vi "Receive Event with Logging.vi"(6 "Global Log Level":T1, 7 "Mediated Actor in":refnum<class "Mediated Actor.lvclass">, 8 "error in (no error)":errorcluster, 11 "Message":refnum<class "Message Interface.lvclass">) -> (0 "error out":errorcluster, 2 "Name":string, 3 "Message out":refnum<class "Message Interface.lvclass">, 5 "Mediated Actor out":refnum<class "Mediated Actor.lvclass">)   [LabVIEW 2016, in "Stream Mediator.lvlib" / "Mediated Actor.lvclass"]
doc: "--\nCopyright © 2017 Composed SystemsI All rights reserved.\n\nAuthor: Jon McBee <jon.mcbee@composed.io>\n\nThis library is provided \"AS IS\" ,WITHOUT WARRANTIES OR\nCONDITIONS OF ANY KIND, either express or implied.\n\nComposed Systems -- composed.io\n\nStream 0.0.1.1\nJon McBee - Composed Systems\nCopyright (c) 2017, Composed Systems"
uses:
  <userlib>/Composed Systems/Stream/Mediator/Classes/Mediated Actor/Mediated Actor.lvclass
  C:/Program Files (x86)/National Instruments/LabVIEW 2016/user.lib/Composed Systems/Stream/Actor/Actor Class/Ancestral Actor.lvclass
  <userlib>/Composed Systems/Stream/Mediator/Classes/Message Interface/Message Interface.lvclass
  <userlib>/Composed Systems/Stream/Log/Application Log/Log Level.ctl
  <userlib>/Composed Systems/Stream/Actor/Actor Class/Ancestral Actor.lvclass/Ancestral Actor.ctl
  <userlib>/Composed Systems/Stream/Mediator/Classes/Message Interface/Message Interface.lvclass/Message Interface.ctl
  <userlib>/Composed Systems/Stream/Log/Global Application Log/Global Application Log.lvclass
  <userlib>/Composed Systems/Stream/Actor/Actor Class/Ancestral Actor.lvclass
  <userlib>/Composed Systems/Stream/Log/Application Log/Application Log.lvclass
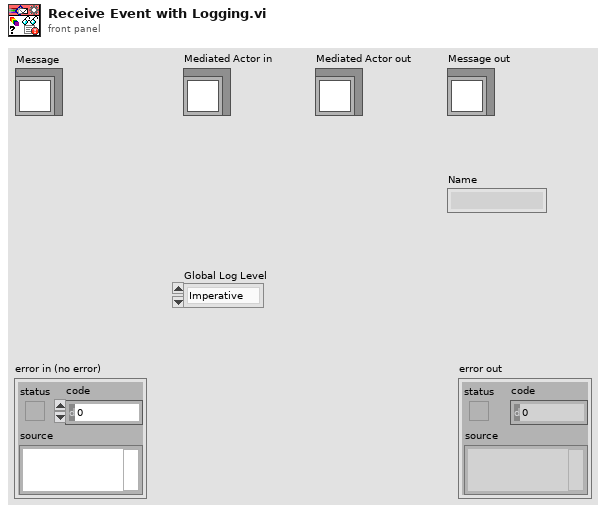
[diagram p1: front panel]
types:
  T1 = typedef "Stream Log.lvlib/Application Log.lvclass/Log Level.ctl" = enum16{"Imperative", "Major", "Minor", "Debug", "Off"}
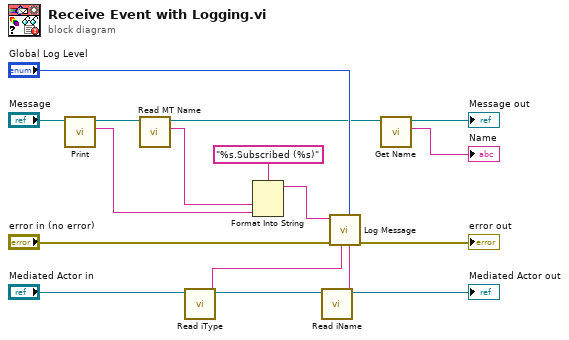
[diagram p0: block diagram]
diagram:
  n1 = call-dynamic "Print.vi"("Message Interface in"="Message") -> ("String"=w1:string, "Message Interface out"=w4:refnum<class "Message Interface.lvclass">)  [unwired: 8 in, 1 out]
  n2 = call <userlib>:"Read MT Name.vi"("Message Interface in"=w4) -> ("MT Name"=w2:string, "Message Interface out"=w3:refnum<class "Message Interface.lvclass">)  [unwired: 9 in]
  n3 = call <userlib>:"Read iType.vi"("Ancestral Actor in"="Mediated Actor in") -> ("iType"=w11:string, "Ancestral Actor out"=w13:refnum<class "Mediated Actor.lvclass">)  [unwired: 8 in, 1 out]
  n4 = Format Into String(format string="%s.Subscribed (%s)", w2, w1) -> (resulting string=w6:string)  [unwired: 2 in, 1 out]
  n5 = call <userlib>:"Read iName.vi"("Ancestral Actor in"=w13) -> ("iName"=w10:string, "Ancestral Actor out"=→"Mediated Actor out":refnum<class "Mediated Actor.lvclass">)  [unwired: 8 in, 1 out]
  n6 = call <userlib>:"Log Message.vi"("Actor Name"=w10, "Level"="Global Log Level", "Actor Type"=w11, "error in (no error)"="error in (no error)", "Message"=w6) -> ("error out"=→"error out":errorcluster)  [unwired: 6 in]
  n7 = call <userlib>:"Get Name.vi"("Message Interface in"=w3) -> ("Name"=→"Name":string, "Message Interface out"=→"Message out":refnum<class "Message Interface.lvclass">)  [unwired: 8 in, 1 out]
